vi "D+andRbXY.vi"(11 "引用句柄输入":T1) -> (3 "Image Out":T1)   [LabVIEW 2014]
uses:
  <vilib>/vision/Image Controls.llb/IMAQ Image.ctl
panel:
  out "error out":errorcluster
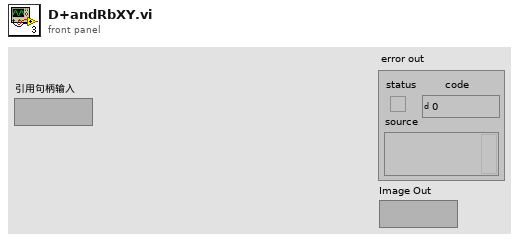
[diagram p1: front panel]
types:
  T1 = typedef "IMAQ Image.ctl" = refnum<image>
  T2 = cluster{"Desired Font (Application)":enum16{"User-specified Font", "Application Font", "System Font", "Dialog Font"}, "[User-specified Font]":cluster{"Font Name":string, "Size":i16, "Strikeout?":bool, "Italic?":bool, "Underline?":bool, "Outline?":bool, "Shadow?":bool, "Bold?":bool, "Rotation Angle":dbl}, "Horizontal Alignment":i16, "Vertical Alignment":i16}
  T3 = cluster{"Left":i32, "Top":i32, "Right":i32, "Bottom":i32}
  T4 = cluster{"Point1 (Pixels)":cluster{"X1":sgl, "Y1":sgl}, "Point2 (Pixels)":cluster{"X2":sgl, "Y2":sgl}}
  T5 = cluster{"Point2 (Pixels)":cluster{"X2":sgl, "Y2":sgl}, cluster{sgl, sgl}}
  T6 = cluster{cluster{sgl, sgl}, "Point2 (Pixels)":cluster{"X2":sgl, "Y2":sgl}}
  T7 = cluster{"Point1 (Pixels)":cluster{"X1":sgl, "Y1":sgl}, cluster{sgl, "Y1":sgl}}
  T8 = cluster{"Point1 (Pixels)":cluster{"X1":sgl, "Y1":sgl}, cluster{sgl, "Y1":sgl}}[]
  T9 = typedef "Image Type" = u32
  T10 = cluster{i32, i32, "X Resolution":i32, "Y Resolution":i32}
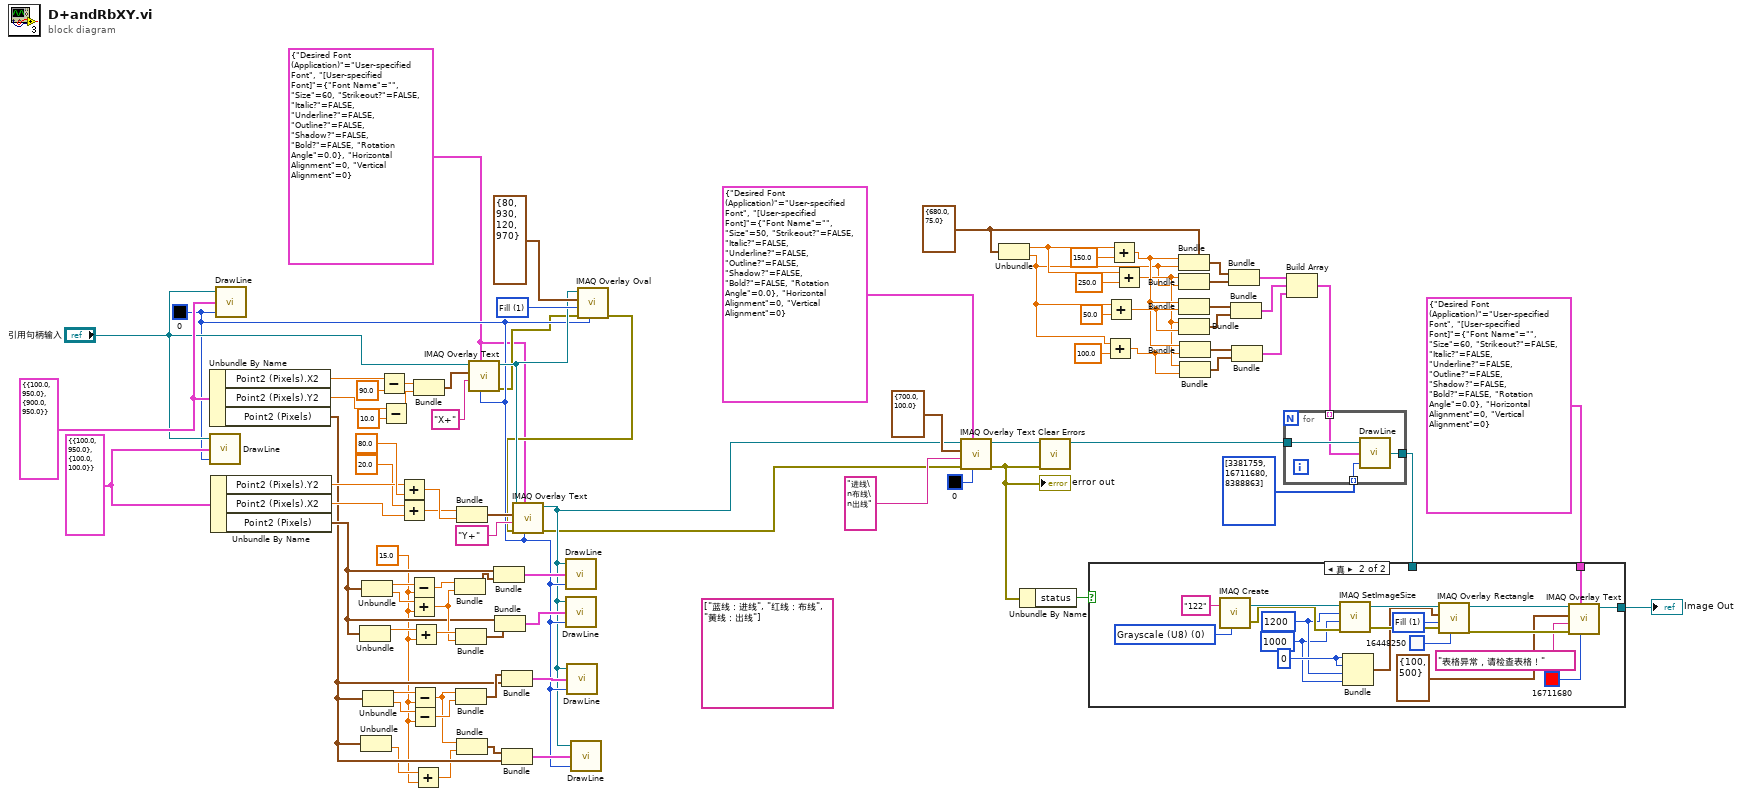
[diagram p0: block diagram]
diagram:
  w15 = sgl 15.0 ("y")
  w41 = u32 1 items=["Frame", "Fill"] ("Drawing Mode (Frame)")
  w55 = cluster{"X1":sgl, "Y1":sgl} {"X1"=680.0, "Y1"=75.0} ("Point1 (Pixels)")
  (unwired) string[] ["蓝线：进线", "红线：布线", "黄线：出线"]
  w13 = u32 0 ("Color")
  w5 = T2 {"Desired Font (Application)"=enum."User-specified Font", "[User-specified Font]"={"Font Name"="", "Size"=60, "Strikeout?"=FALSE, "Italic?"=FALSE, "Underline?"=FALSE, "Outline?"=FALSE, "Shadow?"=FALSE, "Bold?"=FALSE, "Rotation Angle"=0.0}, "Horizontal Alignment"=0, "Vertical Alignment"=0} ("Font, Size & Style")
  w75 = T4 {"Point1 (Pixels)"={"X1"=100.0, "Y1"=950.0}, "Point2 (Pixels)"={"X2"=100.0, "Y2"=100.0}} ("Edge Points")
  w83 = T4 {"Point1 (Pixels)"={"X1"=100.0, "Y1"=950.0}, "Point2 (Pixels)"={"X2"=900.0, "Y2"=950.0}} ("Edge Points")
  n1 = Unbundle By Name(w83) -> ("Point2 (Pixels).X2"=w82:sgl, "Point2 (Pixels).Y2"=w72:sgl, "Point2 (Pixels)"=w19:cluster{"X2":sgl, "Y2":sgl})
  n2 = call "DrawLine.vi"("Color"=w13, "Edge Points"=w75, "img in"="引用句柄输入") -> ()  [unwired: 1 out]
  n3 = Unbundle By Name(w75) -> ("Point2 (Pixels).Y2"=w76:sgl, "Point2 (Pixels).X2"=w73:sgl, "Point2 (Pixels)"=w25:cluster{"X2":sgl, "Y2":sgl})
  n4 = call "DrawLine.vi"("Color"=w13, "Edge Points"=w83, "img in"="引用句柄输入") -> ()  [unwired: 1 out]
  n5 = Unbundle(w25) -> ("X2"=w32:sgl)  [unwired: 1 out]
  n6 = Unbundle(w19) -> ("Y2"=w16:sgl)  [unwired: 1 out]
  n7 = Unbundle(w25) -> ("X2"=w33:sgl, "Y2"=w29:sgl)
  n8 = Unbundle(w19) -> ("X2"=w17:sgl, "Y2"=w21:sgl)
  n9 = Subtract(x=w82, y=sgl 90.0) -> (x-y=w80:sgl)
  n10 = Subtract(x=w72, y=sgl 10.0) -> (x-y=w71:sgl)
  n11 = Add(x=w76, y=sgl 80.0) -> (x+y=w74:sgl)
  n12 = Add(x=sgl 20.0, y=w73) -> (x+y=w39:sgl)
  n13 = Subtract(x=w33, y=w15) -> (x-y=w30:sgl)
  n14 = Add(x=w29, y=w15) -> (x+y=w27:sgl)
  n15 = Subtract(x=w17, y=w15) -> (x-y=w11:sgl)
  n16 = Subtract(x=w21, y=w15) -> (x-y=w22:sgl)
  n17 = Add(x=w32, y=w15) -> (x+y=w28:sgl)
  n18 = Add(x=w16, y=w15) -> (x+y=w14:sgl)
  n19 = Bundle(w80, w71) -> (w79:cluster{sgl, sgl})  [unwired: 1 in]
  n20 = Bundle(w30, w27) -> (w31:cluster{sgl, sgl})  [unwired: 1 in]
  n21 = Bundle(w28, w27) -> (w26:cluster{sgl, sgl})  [unwired: 1 in]
  n22 = Bundle(w11, w22) -> (w20:cluster{sgl, sgl})  [unwired: 1 in]
  n23 = Bundle(w39, w74) -> (w78:cluster{sgl, sgl})  [unwired: 1 in]
  n24 = Bundle(w11, w14) -> (w18:cluster{sgl, sgl})  [unwired: 1 in]
  n25 = call "IMAQ Overlay Text"("Text Color (black)"=w13, "Font, Size & Style"=w5, "String"="X+", "Origin"=w79, "Image"="引用句柄输入") -> ("error out"=w10:errorcluster, "Image Out"=w36:T1)  [unwired: 5 in]
  n26 = Bundle("Point2 (Pixels)"=w25, w31) -> (w35:T5)  [unwired: 1 in]
  n27 = Bundle("Point2 (Pixels)"=w25, w26) -> (w34:T5)  [unwired: 1 in]
  n28 = Bundle(w20, "Point2 (Pixels)"=w19) -> (w24:T6)  [unwired: 1 in]
  n29 = Bundle(w18, "Point2 (Pixels)"=w19) -> (w23:T6)  [unwired: 1 in]
  n30 = call "IMAQ Overlay Oval"("Color"=w13, "error in (no error)"=w10, "Drawing Mode (Frame)"=w41, "Bounding Rectangle"=T3 {"Left"=80, "Top"=930, "Right"=120, "Bottom"=970}, "Image"=w36) -> ("error out"=w9:errorcluster)  [unwired: 5 in, 1 out]
  n31 = call "IMAQ Overlay Text"("Text Color (black)"=w13, "Font, Size & Style"=w5, "error in (no error)"=w9, "String"="Y+", "Origin"=w78, "Image"=w36) -> ("error out"=w8:errorcluster, "Image Out"=w12:T1)  [unwired: 4 in]
  n32 = call "DrawLine.vi"("Color"=w13, "Edge Points"=w35, "img in"=w12) -> ()  [unwired: 1 out]
  n33 = call "DrawLine.vi"("Color"=w13, "Edge Points"=w34, "img in"=w12) -> ()  [unwired: 1 out]
  n34 = call "DrawLine.vi"("Color"=w13, "Edge Points"=w24, "img in"=w12) -> ()  [unwired: 1 out]
  n35 = call "DrawLine.vi"("Color"=w13, "Edge Points"=w23, "img in"=w12) -> ()  [unwired: 1 out]
  n36 = call "IMAQ Overlay Text"("Text Color (black)"=u32 0, "Font, Size & Style"=T2 {"Desired Font (Application)"=enum."User-specified Font", "[User-specified Font]"={"Font Name"="", "Size"=50, "Strikeout?"=FALSE, "Italic?"=FALSE, "Underline?"=FALSE, "Outline?"=FALSE, "Shadow?"=FALSE, "Bold?"=FALSE, "Rotation Angle"=0.0}, "Horizontal Alignment"=0, "Vertical Alignment"=0}, "error in (no error)"=w8, "String"="进线\n布线\n出线", "Origin"=cluster{"X1":sgl, "Y1":sgl} {"X1"=700.0, "Y1"=100.0} ("Point1 (Pixels)"), "Image"=w12) -> ("error out"=w7:errorcluster, "Image Out"=w65:T1)  [unwired: 4 in]
  "error out" <- w7
  n37 = Unbundle(w55) -> ("X1"=w57:sgl, "Y1"=w43:sgl)
  n38 = Unbundle By Name(w7) -> ("status"=w6:bool)
  n39 = call <vilib>:"Clear Errors.vi"("error in (no error)"=w7) -> ()  [unwired: 5 in, 2 out]
  n40 = Add(x=w43, y=sgl 100.0) -> (x+y=w42:sgl)
  n41 = Add(x=w43, y=sgl 50.0) -> (x+y=w50:sgl)
  n42 = Add(x=w57, y=sgl 150.0) -> (x+y=w46:sgl)
  n43 = Add(x=w57, y=sgl 250.0) -> (x+y=w45:sgl)
  n44 = Bundle(cluster=w55, "X1"=w46, "Y1"=w43) -> (w62:cluster{"X1":sgl, "Y1":sgl})
  n45 = Bundle(w45, "Y1"=w43) -> (w56:cluster{sgl, "Y1":sgl})  [unwired: 1 in]
  n46 = Bundle(w46, w50) -> (w53:cluster{sgl, sgl})  [unwired: 1 in]
  n47 = Bundle(w45, w50) -> (w51:cluster{sgl, sgl})  [unwired: 1 in]
  n48 = Bundle(w46, w42) -> (w47:cluster{sgl, sgl})  [unwired: 1 in]
  n49 = Bundle(w45, w42) -> (w49:cluster{sgl, sgl})  [unwired: 1 in]
  n50 = Bundle("Point1 (Pixels)"=w62, w56) -> (w63:T7)  [unwired: 1 in]
  n51 = Bundle(w53, w51) -> (w52:cluster{cluster{sgl, sgl}, cluster{sgl, sgl}})  [unwired: 1 in]
  n52 = Bundle(w47, w49) -> (w48:cluster{cluster{sgl, sgl}, cluster{sgl, sgl}})  [unwired: 1 in]
  n53 = Build Array(w63, w52, w48) -> (w61:T8)
  n54 = for {
    tunnel: w65 -> [w87]
    tunnel: w61 -> [w86] mode=indexing
    tunnel: u32[] [3381759, 16711680, 8388863] -> [w85] mode=indexing
    tunnel: [w84] -> w2
    n55 = call "DrawLine.vi"("Color"=w85, "Edge Points"=w86, "img in"=w87) -> ("Image Out"=w84:T1)
  }
  n56 = case shown="真" w6 {
    tunnel: T2 {"Desired Font (Application)"=enum."User-specified Font", "[User-specified Font]"={"Font Name"="", "Size"=60, "Strikeout?"=FALSE, "Italic?"=FALSE, "Underline?"=FALSE, "Outline?"=FALSE, "Shadow?"=FALSE, "Bold?"=FALSE, "Rotation Angle"=0.0}, "Horizontal Alignment"=0, "Vertical Alignment"=0} ("Font, Size & Style") -> [_ w97]
    tunnel: [w88 w90] -> w1
    tunnel: w2 -> [w88 _]
    frame False {
    }
    frame True {
      w94 = 0
      w103 = u32 1 items=["Frame", "Fill", "Highlight"] ("Drawing Mode (Frame)")
      w91 = 1000 ("Y Resolution")
      w92 = 1200 ("X Resolution")
      w106 = T9 0 items=["Grayscale (U8)", "Grayscale (I16)", "Grayscale (SGL)", "Complex (CSG)", "RGB (U32)", "HSL (U32)", "RGB (U64)", "Grayscale (U16)"] ("Image Type")
      n57 = call "IMAQ Create"("Image Name"="122", "Image Type"=w106) -> ("New Image"=w107:T1, "error out"=w104:errorcluster)  [unwired: 3 in]
      n58 = call "IMAQ SetImageSize"("error in (no error)"=w104, "Y Resolution"=w91, "X Resolution"=w92, "Image"=w107) -> ("error out"=w102:errorcluster, "Image Out"=w101:T1)  [unwired: 1 in]
      n59 = Bundle(w94, w94, "X Resolution"=w92, "Y Resolution"=w91) -> (w93:T10)  [unwired: 1 in]
      n60 = call "IMAQ Overlay Rectangle"("Color"=u32 16448250, "error in (no error)"=w102, "Drawing Mode (Frame)"=w103, "Rectangle"=w93, "Image"=w101) -> ("error out"=w98:errorcluster, "Image Out"=w99:T1)  [unwired: 5 in]
      n61 = call "IMAQ Overlay Text"("Text Color (black)"=u32 16711680, "Font, Size & Style"=w97, "error in (no error)"=w98, "String"="表格异常，请检查表格！", "Origin"=cluster{"X":i32, "Y":i32} {"X"=100, "Y"=500}, "Image"=w99) -> ("Image Out"=w90:T1)  [unwired: 4 in, 1 out]
    }
  }
  "Image Out" <- w1
